vi "Init.vi"(10 "Event":refnum<class "Event.lvclass">) -> (3 "Last Ack Created Event Msg Strategy out":refnum<class "Last Ack Created Event Msg Strategy.lvclass">)   [LabVIEW 2021, in "jettl.lvlib" / "Last Ack Created Event Msg Strategy.lvlib" / "Last Ack Created Event Msg Strategy.lvclass"]
uses:
  Last Ack Created Event Msg Strategy.lvclass
  Event/Event.lvclass
  Last Ack Created Event Msg Strategy.lvclass/Last Ack Created Event Msg Strategy.ctl
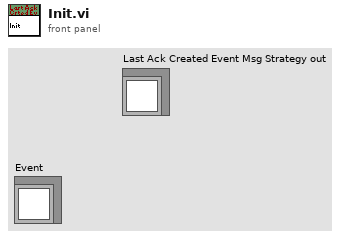
[diagram p1: front panel]
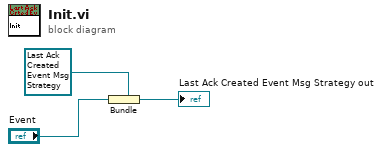
[diagram p0: block diagram]
diagram:
  n1 = Bundle(cluster=refnum<class "Last Ack Created Event Msg Strategy.lvclass"> refnum ("Event Last Ack Msg out"), "Event") -> (→"Last Ack Created Event Msg Strategy out":refnum<class "Last Ack Created Event Msg Strategy.lvclass">)
